vi "licorfpgainit.vi"() -> (0 "FPGA VI Reference Out":refnum<k20>)   [LabVIEW 2010]
uses:
  <vilib>/userDefined/High Color/nirio_resource_hc.ctl
  <vilib>/rvi/interface/nirviOpenFPGA/nirviOpenFPGA.xnode
  <vilib>/rvi/interface/nirviMethod/nirviMethod.xnode
  <vilib>/LabVIEW Targets/FPGA/cRIO/shared/nicrio_ModuleControls/nicrio_cRIO-9871_FlowControlEnum.ctl
  <vilib>/LabVIEW Targets/FPGA/cRIO/shared/nicrio_ModuleControls/nicrio_cRIO-9871_StopBitsEnum.ctl
  <vilib>/LabVIEW Targets/FPGA/cRIO/shared/nicrio_ModuleControls/nicrio_cRIO-9871_ParityEnum.ctl
  <vilib>/LabVIEW Targets/FPGA/cRIO/shared/nicrio_ModuleControls/nicrio_cRIO-9871_DataBitsEnum.ctl
  <vilib>/LabVIEW Targets/FPGA/cRIO/shared/nicrio_ModuleControls/nicrio_cRIO-9871_BaudRateEnum.ctl
  <vilib>/rvi/interface/nirviReadWriteControl/nirviReadWriteControl.xnode
  <vilib>/rvi/errors/niLvFpgaWhatHappensToTopLevelVI.ctl
  <vilib>/rvi/interface/common/niFpgaNodeNameForErrorReporting.ctl
  <vilib>/rvi/errors/niLvFpgaAdjustHostInterfaceError.vi
  C:/Users/HAGAR-IV/Desktop/Zeugs/markus/version feb 2012/FPGA Bitfiles/pertrasgcfpga2_FPGATarget_FPGA-Programm-10_16368CB6.lvbitx
  C:/Users/HAGAR-IV/Desktop/Zeugs/Johnny/pertrasgc fpga/FPGA-Programm-10-14.vi
  NiFpgaLv.dll
  <vilib>/Utility/error.llb/Error Cluster From Error Code.vi
  <vilib>/RVI Host/nirviSupport.llb/nirviErrorClusterFromErrorCode.vi
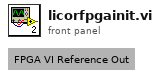
[diagram p1: front panel]
types:
  T1 = cluster{"ServoTrap1kalt":bool, "Servo1WarmHigh(us)":u32, "Servo1KaltHigh(us)":u32, "ServoTrap2kalt":bool, "Servo2WarmHigh(us)":u32, "Servo2KaltHigh(us)":u32}
  T2 = cluster{"PIDMach1":cluster{"proportional gain (Kc)":fxp<+/-,16,8>, "integral gain (Kc*Ts/Ti)":fxp<+/-,16,8>, "derivative gain (Kc*Td/Ts)":fxp<+/-,16,8>}, "Umax[V]Mach1":fxp<+/-,16,4>, "Heizen?Mach1":bool, "USetp[V]Mach1":fxp<+/-,16,4>, "PIDMach2":cluster{"proportional gain (Kc)":fxp<+/-,16,8>, "integral gain (Kc*Ts/Ti)":fxp<+/-,16,8>, "derivative gain (Kc*Td/Ts)":fxp<+/-,16,8>}, "Umax[V]Mach2":fxp<+/-,16,4>, "Heizen?Mach2":bool, "USetp[V]Mach2":fxp<+/-,16,4>}
  T3 = cluster{"PIDTrap1":cluster{"proportional gain (Kc)":fxp<+/-,16,8>, "integral gain (Kc*Ts/Ti)":fxp<+/-,16,8>, "derivative gain (Kc*Td/Ts)":fxp<+/-,16,8>}, "UTempMaxTrap1":fxp<+/-,16,4>, "UWidrMaxTrap1":fxp<+/-,16,4>, "Heizen?Trap1":bool, "UTempSPTrap1":fxp<+/-,16,4>}
  T4 = cluster{"Bronkhorst1":bool, "Bronkhorst1 ":u16, "MainCol1":bool, "MainCol1":u16, "MainCol2":bool, "MainCol2":u16, "Bronkhorst2":bool, "Bronkhorst2":u16, "Oven":bool, "Oven":u16, "T-Line":bool, "T-Line":u16}
  T5 = cluster{"Mod6/DIO0":bool, "Mod6/DIO3":bool, "Mod6/DIO4":bool, "Mod6/DIO5":bool, "Mod6/DIO6":bool, "Mod6/DIO7":bool, "Mod6/DIO8":bool, "Mod6/DIO9":bool, "Mod6/DIO10":bool, "Mod6/DIO11":bool, "Mod6/DIO12":bool, "Mod6/DIO13":bool, "Mod6/DIO14":bool, "Mod6/DIO15":bool, "Mod6/DIO16":bool, "Mod6/DIO17":bool, "Mod6/DIO18":bool, "Mod6/DIO19":bool, "Mod6/DIO20":bool, "Mod6/DIO21":bool, "Mod6/DIO22":bool, "Mod6/DIO23":bool, "Mod6/DIO24":bool, "Mod6/DIO25":bool, "Mod6/DIO26":bool, "Mod6/DIO27":bool, "Mod6/DIO28":bool, "Mod6/DIO29":bool, "Mod6/DIO30":bool, "Mod6/DIO31":bool}
  T6 = cluster{"Mod5/DIO5":bool, "Mod5/DIO6":bool, "Mod5/DIO7":bool, "Mod5/DIO10":bool, "Mod5/DIO11":bool, "Mod5/DIO14":bool, "Mod5/DIO15":bool, "Mod5/DIO16":bool, "Mod5/DIO17":bool, "Mod5/DIO18":bool, "Mod5/DIO20":bool, "Mod5/DIO23":bool, "Mod5/DIO25":bool, "Mod5/DIO26":bool, "Mod5/DIO27":bool, "Mod5/DIO28":bool, "Mod5/DIO29":bool, "Mod5/DIO30":bool}
  T7 = typedef "nicrio_cRIO-9871_BaudRateEnum.ctl" = enum16{"75 bps", "110 bps", "134 bps", "150 bps", "300 bps", "600 bps", "1200 bps", "1800 bps", "2400 bps", "4800 bps", "7200 bps", "9600 bps", "14.4 kbps", "19.2 kbps", "28.8 kbps", "38.4 kbps", "57.6 kbps", "115.2 kbps", "230.4 kbps", "460.8 kbps", "921.6 kbps"}
  T8 = typedef "nicrio_cRIO-9871_DataBitsEnum.ctl" = enum8{"5", "6", "7", "8"}
  T9 = typedef "nicrio_cRIO-9871_ParityEnum.ctl" = enum8{"None", "Odd", "Even", "Mark", "Space"}
  T10 = typedef "nicrio_cRIO-9871_StopBitsEnum.ctl" = enum8{"1", "1.5", "2"}
  T11 = typedef "nicrio_cRIO-9871_FlowControlEnum.ctl" = enum8{"None", "Software (XON / XOFF)", "Hardware (RTS / CTS)"}
  T12 = cluster{"Mod7/Port1":cluster{"Baud Rate":T7, "Data Bits":T8, "Parity":T9, "Stop Bits":T10, "Flow Control":T11}, "Mod7/Port2":cluster{"Baud Rate":T7, "Data Bits":T8, "Parity":T9, "Stop Bits":T10, "Flow Control":T11}, "Mod7/Port3":cluster{"Baud Rate":T7, "Data Bits":T8, "Parity":T9, "Stop Bits":T10, "Flow Control":T11}, "Mod7/Port4":cluster{"Baud Rate":T7, "Data Bits":T8, "Parity":T9, "Stop Bits":T10, "Flow Control":T11}, "Mod8/Port1":cluster{"Baud Rate":T7, "Data Bits":T8, "Parity":T9, "Stop Bits":T10, "Flow Control":T11}, "Mod8/Port2":cluster{"Baud Rate":T7, "Data Bits":T8, "Parity":T9, "Stop Bits":T10, "Flow Control":T11}, "Mod8/Port3":cluster{"Baud Rate":T7, "Data Bits":T8, "Parity":T9, "Stop Bits":T10, "Flow Control":T11}, "Mod8/Port4":cluster{"Baud Rate":T7, "Data Bits":T8, "Parity":T9, "Stop Bits":T10, "Flow Control":T11}}
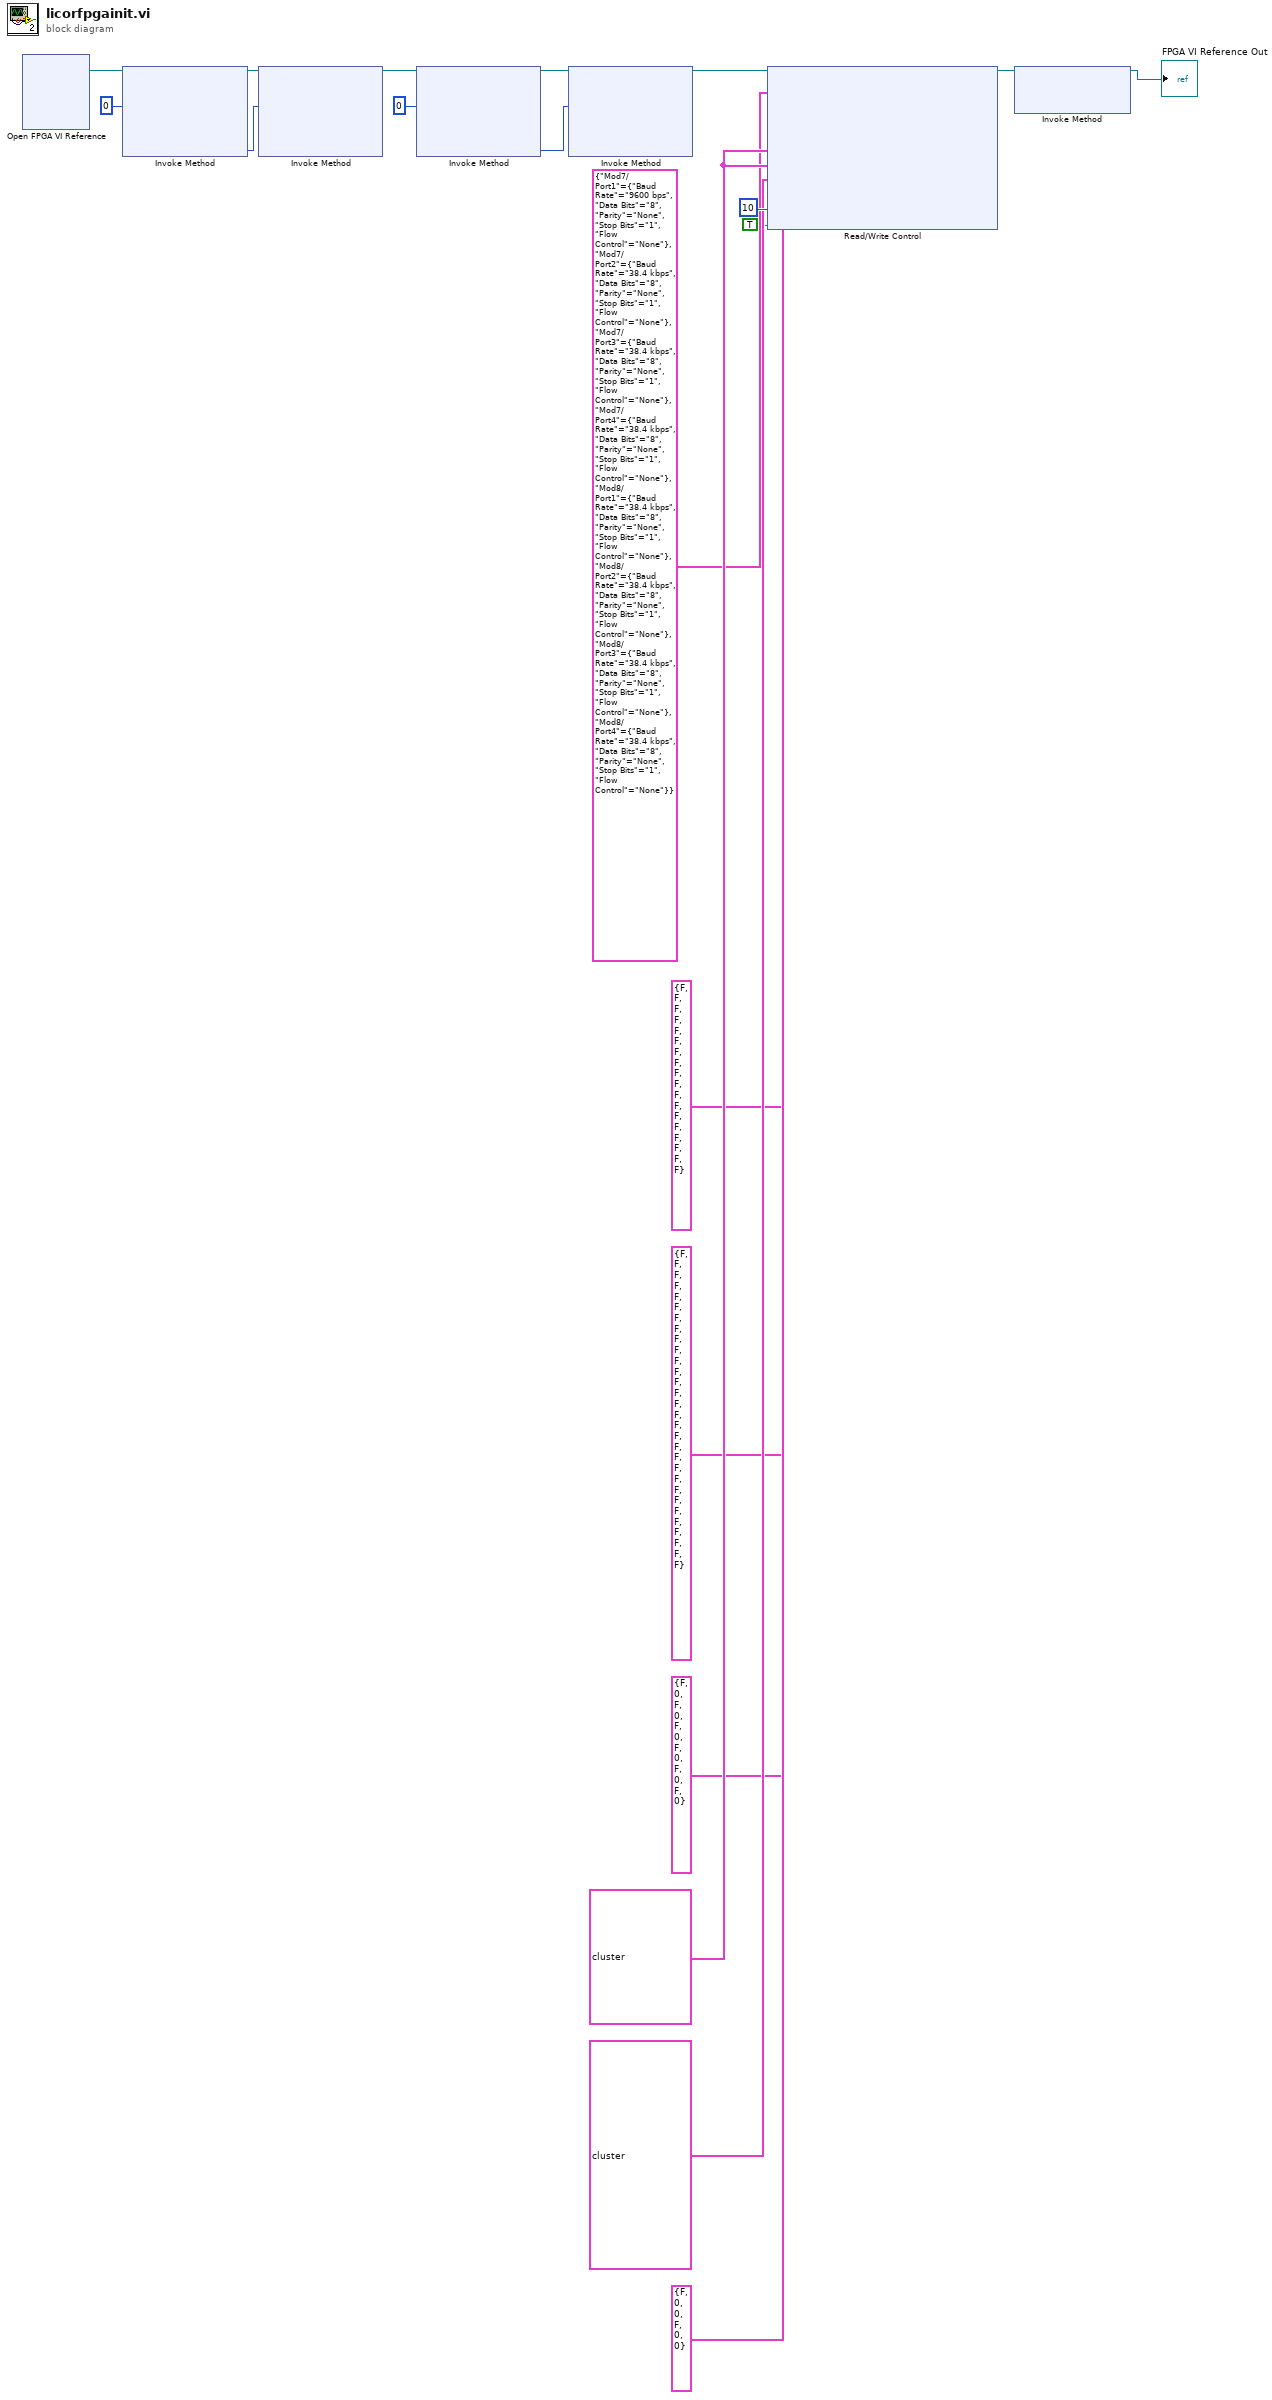
[diagram p0: block diagram]
diagram:
  w16 = T3 {"PIDTrap1"={"proportional gain (Kc)"=0.0, "integral gain (Kc*Ts/Ti)"=0.0, "derivative gain (Kc*Td/Ts)"=0.0}, "UTempMaxTrap1"=0.0, "UWidrMaxTrap1"=0.0, "Heizen?Trap1"=FALSE, "UTempSPTrap1"=0.0} ("Trap1")
  n1 = xnode "Open FPGA VI Reference"() -> ("FPGA VI Reference Out"=w3:refnum<k20>)  [unwired: 2 in, 1 out]
  n2 = xnode "Invoke Method"("FPGA VI Reference In"=w3, "Number of Elements"=u32 0) -> ("FPGA VI Reference Out"=w5:refnum<k20>, "Elements Remaining"=w6:u32)  [unwired: 2 in, 2 out]
  n3 = xnode "Invoke Method"("FPGA VI Reference In"=w5, "Number of Elements"=w6) -> ("FPGA VI Reference Out"=w7:refnum<k20>)  [unwired: 2 in, 3 out]
  n4 = xnode "Invoke Method"("FPGA VI Reference In"=w7, "Number of Elements"=u32 0) -> ("FPGA VI Reference Out"=w9:refnum<k20>, "Elements Remaining"=w10:u32)  [unwired: 2 in, 2 out]
  n5 = xnode "Invoke Method"("FPGA VI Reference In"=w9, "Number of Elements"=w10) -> ("FPGA VI Reference Out"=w11:refnum<k20>)  [unwired: 2 in, 3 out]
  n6 = xnode "Read/Write Control"("FPGA VI Reference In"=w11, "KonfigSeriell"=T12 {"Mod7/Port1"={"Baud Rate"=enum."9600 bps", "Data Bits"=enum."8", "Parity"=enum."None", "Stop Bits"=enum."1", "Flow Control"=enum."None"}, "Mod7/Port2"={"Baud Rate"=enum."38.4 kbps", "Data Bits"=enum."8", "Parity"=enum."None", "Stop Bits"=enum."1", "Flow Control"=enum."None"}, "Mod7/Port3"={"Baud Rate"=enum."38.4 kbps", "Data Bits"=enum."8", "Parity"=enum."None", "Stop Bits"=enum."1", "Flow Control"=enum."None"}, "Mod7/Port4"={"Baud Rate"=enum."38.4 kbps", "Data Bits"=enum."8", "Parity"=enum."None", "Stop Bits"=enum."1", "Flow Control"=enum."None"}, "Mod8/Port1"={"Baud Rate"=enum."38.4 kbps", "Data Bits"=enum."8", "Parity"=enum."None", "Stop Bits"=enum."1", "Flow Control"=enum."None"}, "Mod8/Port2"={"Baud Rate"=enum."38.4 kbps", "Data Bits"=enum."8", "Parity"=enum."None", "Stop Bits"=enum."1", "Flow Control"=enum."None"}, "Mod8/Port3"={"Baud Rate"=enum."38.4 kbps", "Data Bits"=enum."8", "Parity"=enum."None", "Stop Bits"=enum."1", "Flow Control"=enum."None"}, "Mod8/Port4"={"Baud Rate"=enum."38.4 kbps", "Data Bits"=enum."8", "Parity"=enum."None", "Stop Bits"=enum."1", "Flow Control"=enum."None"}}, "Mod5/DIOs"=T6 {"Mod5/DIO5"=FALSE, "Mod5/DIO6"=FALSE, "Mod5/DIO7"=FALSE, "Mod5/DIO10"=FALSE, "Mod5/DIO11"=FALSE, "Mod5/DIO14"=FALSE, "Mod5/DIO15"=FALSE, "Mod5/DIO16"=FALSE, "Mod5/DIO17"=FALSE, "Mod5/DIO18"=FALSE, "Mod5/DIO20"=FALSE, "Mod5/DIO23"=FALSE, "Mod5/DIO25"=FALSE, "Mod5/DIO26"=FALSE, "Mod5/DIO27"=FALSE, "Mod5/DIO28"=FALSE, "Mod5/DIO29"=FALSE, "Mod5/DIO30"=FALSE}, "Mod6/DIOs"=T5 {"Mod6/DIO0"=FALSE, "Mod6/DIO3"=FALSE, "Mod6/DIO4"=FALSE, "Mod6/DIO5"=FALSE, "Mod6/DIO6"=FALSE, "Mod6/DIO7"=FALSE, "Mod6/DIO8"=FALSE, "Mod6/DIO9"=FALSE, "Mod6/DIO10"=FALSE, "Mod6/DIO11"=FALSE, "Mod6/DIO12"=FALSE, "Mod6/DIO13"=FALSE, "Mod6/DIO14"=FALSE, "Mod6/DIO15"=FALSE, "Mod6/DIO16"=FALSE, "Mod6/DIO17"=FALSE, "Mod6/DIO18"=FALSE, "Mod6/DIO19"=FALSE, "Mod6/DIO20"=FALSE, "Mod6/DIO21"=FALSE, "Mod6/DIO22"=FALSE, "Mod6/DIO23"=FALSE, "Mod6/DIO24"=FALSE, "Mod6/DIO25"=FALSE, "Mod6/DIO26"=FALSE, "Mod6/DIO27"=FALSE, "Mod6/DIO28"=FALSE, "Mod6/DIO29"=FALSE, "Mod6/DIO30"=FALSE, "Mod6/DIO31"=FALSE}, "LH Heizen? Pulse (us)"=T4 {"Bronkhorst1"=FALSE, "Bronkhorst1 "=0, "MainCol1"=FALSE, "MainCol1"=0, "MainCol2"=FALSE, "MainCol2"=0, "Bronkhorst2"=FALSE, "Bronkhorst2"=0, "Oven"=FALSE, "Oven"=0, "T-Line"=FALSE, "T-Line"=0}, "Trap1"=w16, "Trap2"=w16, "Machs"=T2 {"PIDMach1"={"proportional gain (Kc)"=0.0, "integral gain (Kc*Ts/Ti)"=0.0, "derivative gain (Kc*Td/Ts)"=0.0}, "Umax[V]Mach1"=0.0, "Heizen?Mach1"=FALSE, "USetp[V]Mach1"=0.0, "PIDMach2"={"proportional gain (Kc)"=0.0, "integral gain (Kc*Ts/Ti)"=0.0, "derivative gain (Kc*Td/Ts)"=0.0}, "Umax[V]Mach2"=0.0, "Heizen?Mach2"=FALSE, "USetp[V]Mach2"=0.0}, "Servos kalt? WarmHigh (us) KaltHigh (us)"=T1 {"ServoTrap1kalt"=FALSE, "Servo1WarmHigh(us)"=0, "Servo1KaltHigh(us)"=0, "ServoTrap2kalt"=FALSE, "Servo2WarmHigh(us)"=0, "Servo2KaltHigh(us)"=0}, "ServosPeriode(us)"=u32 10, "FIFO leer"=TRUE) -> ("FPGA VI Reference Out"=w20:refnum<k20>)  [unwired: 1 in, 1 out]
  n7 = xnode "Invoke Method"("FPGA VI Reference In"=w20) -> ("FPGA VI Reference Out"=→"FPGA VI Reference Out":refnum<k20>)  [unwired: 2 in, 1 out]
